vi "CRYReport Pic Save VI Image.vi"(9 "sData":string, 10 "pVIRef":refnum<vi>, 11 "cFrame":T1) -> (1 "sData_Out":string, 3 "cFrame_Out":T1)   [LabVIEW 2013]
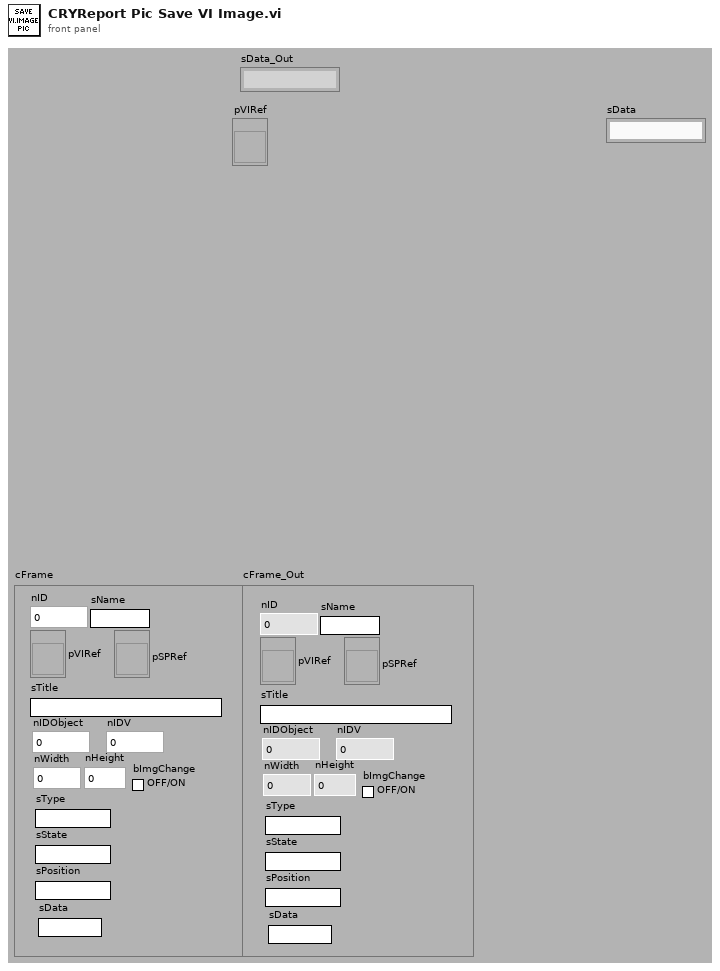
[diagram p1: front panel]
types:
  T1 = cluster{"nID":i16, "sName":string, "pVIRef":refnum<vi>, "pSPRef":refnum<vi>, "sTitle":string, "nIDObject":i16, "nIDV":i16, "nWidth":i16, "nHeight":i16, "bImgChange":bool, "sType":string, "sState":string, "sPosition":string, "sData":string}
  T2 = typedef "imagedata.ctl" = cluster{"image type":i32, "image depth":i32, "image":u8[], "mask":u8[], "colors":u32[], "Rectangle":cluster{"left":i16, "top":i16, "right":i16, "bottom":i16}}
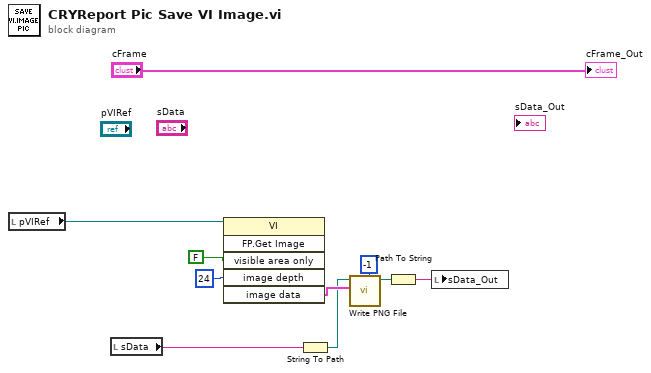
[diagram p0: block diagram]
diagram:
  n1 = local read "pVIRef"() -> (w1:refnum<vi>)
  n2 = local read "sData"() -> (w3:string)
  n3 = invoke class="VI" method="FP.Get Image"(reference=w1, "visible area only"=FALSE ("Visible Area Only"), "image depth"=24 ("Image Depth")) -> ("image data"=w7:T2)  [unwired: 3 in, 5 out]
  n4 = String To Path(string=w3) -> (path=w6:path)
  n5 = call <vilib>:"Write PNG File.vi"("compression (default)"=-1, "image data"=w7, "path to PNG file"=w6) -> ("path"=w5:path)  [unwired: 1 in, 7 out]
  n6 = Path To String(path=w5) -> (string=w4:string)
  n7 = local write "sData_Out"(w4) -> ()
  "cFrame_Out" <- "cFrame"
